vi "Keith 7001 Close.vi"(1 "error in":T1, 2 "type of dialog (OK msg:1)":i32(ring)=1 items=["no dialog", "OK message", "continue or stop message"], 3 "GPIB address":string) -> (0 "error out":T1)   [LabVIEW 2019]
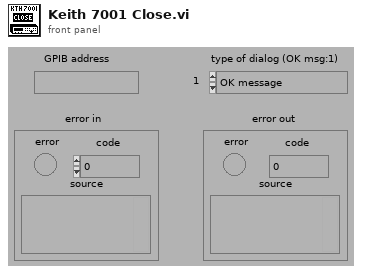
[diagram p1: front panel]
types:
  T1 = cluster{"error":bool, "code":i32, "source":string}
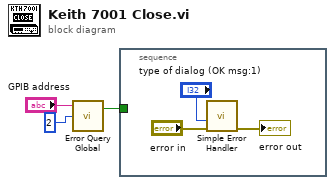
[diagram p0: block diagram]
diagram:
  n1 = call "Error Query Global.vi"("mode (0:read value)"=u16 2, "GPIB address"="GPIB address") -> ("address already present?"=w1:bool)  [unwired: 1 in, 1 out]
  n2 = stacked-sequence {
    tunnel: w1 -> [_]
    frame #0 {
      n3 = call <vilib>:"Simple Error Handler.vi"("type of dialog (OK msg:1)"="type of dialog (OK msg:1)", "error in (no error)"="error in") -> ("error out"=→"error out":errorcluster)  [unwired: 3 in, 4 out]
    }
  }
